vi "manuitest.vi"() -> ()   [LabVIEW 2013, in "VI-Test.lvlib"]
uses:
  lib/VI-Test.lvlib
  classes/Tests/TestInterface/TestInterface.lvclass
  classes/Devices/emTestCWS500N/EMTestCWS500N.lvclass
  classes/Devices/CEG4500/CEG4500.lvclass
panel:
  out "error out 2":errorcluster caption="Fehler (Ausgang)"
  out "error out":errorcluster caption="Fehler (Ausgang)"
  out "TestInterface Ausgang 2":refnum<class "TestInterface.lvclass"> caption="DNL_LabVIEW Object out"
  out "Parameters":u32[](array[numeric])
  out "TestInterface Ausgang":refnum<class "TestInterface.lvclass"> caption="DNL_LabVIEW Object out"
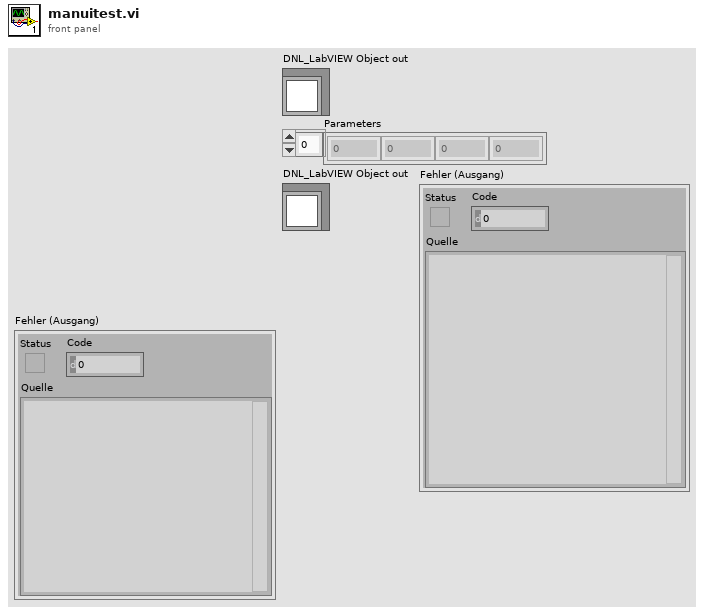
[diagram p1: front panel]
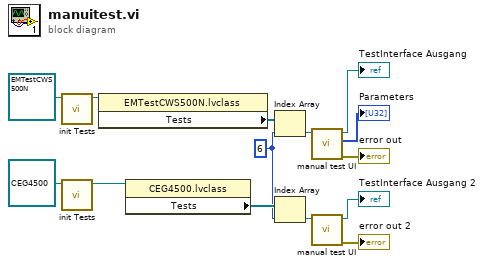
[diagram p0: block diagram]
diagram:
  w7 = 6 ("index")
  n1 = call-dynamic "init Tests.vi"("EMTestCWS500N Eingang"=refnum<class "EMTestCWS500N.lvclass"> refnum) -> ("EMTestCWS500N Ausgang"=w14:refnum<class "EMTestCWS500N.lvclass">)  [unwired: 9 in, 1 out]
  n2 = call-dynamic "init Tests.vi"("CEG4500 Eingang"=refnum<class "CEG4500.lvclass"> refnum ("CEG4500.lvclass")) -> ("CEG4500 Ausgang"=w10:refnum<class "CEG4500.lvclass">)  [unwired: 9 in, 1 out]
  n3 = property class="EMTestCWS500N.lvclass"(reference=w14) -> ("Tests"=w12:refnum<class "TestInterface.lvclass">[])  [unwired: 1 in, 2 out]
  n4 = property class="CEG4500.lvclass"(reference=w10) -> ("Tests"=w9:refnum<class "TestInterface.lvclass">[])  [unwired: 1 in, 2 out]
  n5 = Index Array(array=w12, index=w7) -> (element=w5:refnum<class "TestInterface.lvclass">)
  n6 = Index Array(array=w9, index=w7) -> (element=w8:refnum<class "TestInterface.lvclass">)
  n7 = call-dynamic "manual test UI.vi"("TestInterface Eingang"=w5) -> ("error out"=→"error out":errorcluster, "Parameters"=→"Parameters":u32[], "TestInterface Ausgang"=→"TestInterface Ausgang":refnum<class "TestInterface.lvclass">)  [unwired: 7 in, 1 out]
  n8 = call-dynamic "manual test UI.vi"("TestInterface Eingang"=w8) -> ("error out"=→"error out 2":errorcluster, "TestInterface Ausgang"=→"TestInterface Ausgang 2":refnum<class "TestInterface.lvclass">)  [unwired: 7 in, 2 out]
